vi "AT Get Bool A.vi"(8 "error in (no error)":errorcluster, 10 "Feature":string, 11 "Handle":i32) -> (0 "error out":errorcluster, 2 "Value":bool, 3 "Status":i32)   [LabVIEW 2009]
doc: "Get Bool\n\nOutput:\n I32 Status\n Bool Value\n\nInput:\n I32 Handle\n String Feature\n\nThis function will return the current value of the specified boolean feature. If a value of AT_FALSE is returned then the feature is currently set to false. If a value of AT_TRUE is returned then the feature is currently set to true. An error will be returned if the feature is currently not readable, not a boolean feature or is not implemented by the camera."
uses:
  atcoreA.dll
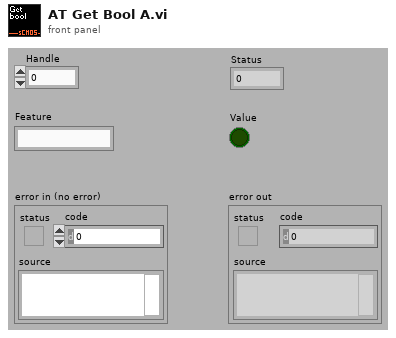
[diagram p1: front panel]
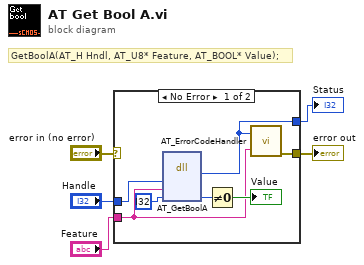
[diagram p0: block diagram]
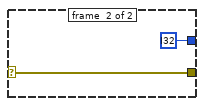
[diagram p2: hidden frame]
diagram:
  # "GetBoolA(AT_H Hndl, AT_U8* Feature, AT_BOOL* Value);"
  n1 = case shown="No Error" "error in (no error)" {
    selector: "error in (no error)" -> [_ w13]
    tunnel: [w6 i32 ?] -> w5
    tunnel: "Handle" -> [w12 _]
    tunnel: "Feature" -> [w7 _]
    tunnel: [w8 w13] -> w1
    frame #0 {
      n2 = dll-call lib="atcoreA.dll" fn="AT_GetBoolA"("Handle"=w12, "Feature"=w7, "Value"=i32 ?) -> ("Status"=w6:i32, "Value"=w9:i32)  [unwired: 5 in, 2 out]
      n3 = Not Equal To 0?(x=w9) -> (x != 0?=→"Value":bool)
      n4 = call "AT_ErrorCodeHandler.vi"("Error"=w6, "Feature Name"=w7) -> ("error out"=w8:errorcluster)  [unwired: 5 in]
    }
    frame #1 {
    }
  }
  "Status" <- w5
  "error out" <- w1
